vi "http write header to string.vi"(11 "application request":T1) -> (3 "header string":string)   [LabVIEW 2013, in "Basic HTTP server.lvclass"]
uses:
  Basic HTTP server.lvclass
  http response.ctl
  http response packet type.ctl
  HTTP headers/http header data.ctl
  HTTP headers/http headers.lvlib
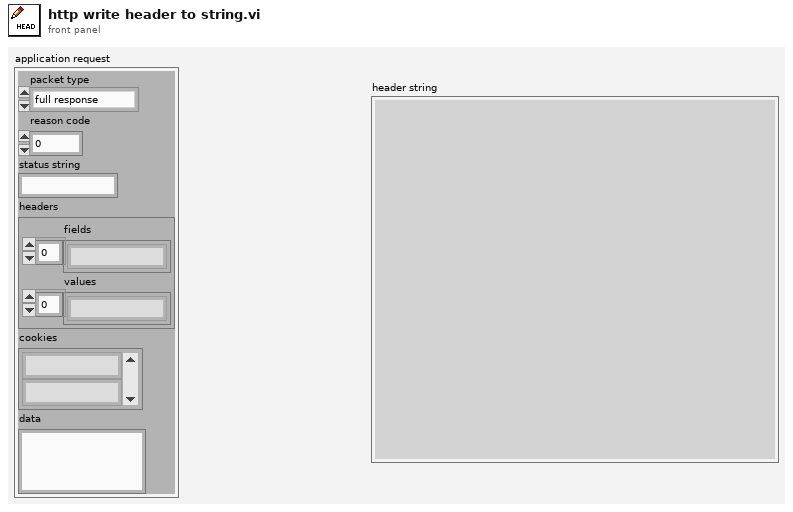
[diagram p1: front panel]
types:
  T1 = typedef "Basic HTTP server.lvclass/http response.ctl" = cluster{"packet type":T2, "reason code":u16, "status string":string, "headers":T3, "cookies":string[], "data":string}
  T2 = typedef "Basic HTTP server.lvclass/http response packet type.ctl" = enum16{"full response", "header only", "data only", "last data"}
  T3 = typedef "http headers.lvlib/http header data.ctl" = cluster{"fields":string[], "values":string[]}
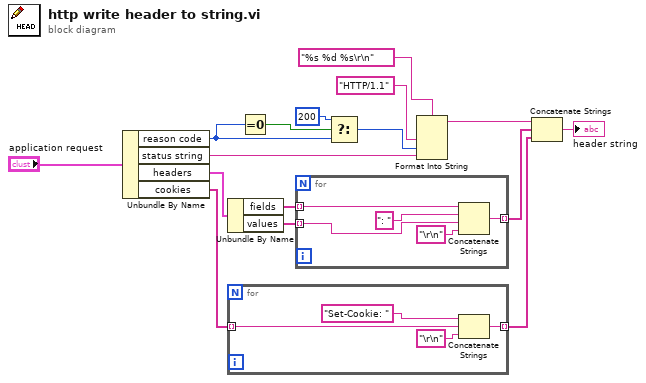
[diagram p0: block diagram]
diagram:
  n1 = Unbundle By Name("application request") -> ("reason code"=w9:u16, "status string"=w14:string, "headers"=w7:T3, "cookies"=w16:string[])
  n2 = Unbundle By Name(w7) -> ("fields"=w6:string[], "values"=w5:string[])
  n3 = for {
    tunnel: w16 -> [w18] mode=indexing
    tunnel: [w17] -> w2 mode=indexing
    n4 = Concatenate Strings("Set-Cookie: " ("string"), w18, "\r\n" ("format string")) -> (w17:string)
  }
  n5 = Equal To 0?(x=w9) -> (x = 0?=w11:bool)
  n6 = for {
    tunnel: w6 -> [w25] mode=indexing
    tunnel: w5 -> [w23] mode=indexing
    tunnel: [w21] -> w3 mode=indexing
    n7 = Concatenate Strings(w25, ": " ("string"), w23, "\r\n" ("format string")) -> (w21:string)
  }
  n8 = Select(t=u16 200, s=w11, f=w9) -> (s? t:f=w8:u16)
  n9 = Format Into String(format string="%s %d %s\r\n", "HTTP/1.1" ("input 1"), w8, w14) -> (resulting string=w4:string)  [unwired: 2 in, 1 out]
  n10 = Concatenate Strings(w4, w3, w2) -> (→"header string":string)
